vi "Init.vi"(8 "error in (no error)":errorcluster, 9 "SA Pin":string, 10 "Measurement Name":string) -> (0 "error out":errorcluster, 3 "GSM_ModAcc_out":refnum<class "GSM_ModAcc.lvclass">)   [LabVIEW 2016, in "SeqAuto Evaluations.lvlib" / "GSM_ModAcc.lvclass"]
uses:
  GSM_ModAcc.lvclass
  C:/Sequence Automation/Plugins/SeqAuto IEvaluation.lvlibp/SeqAuto IEvaluation.lvclass
  GSM_ModAcc.lvclass/GSM_ModAcc.ctl
  Plugins/SeqAuto IEvaluation.lvlibp/Write Measurement Name.vi
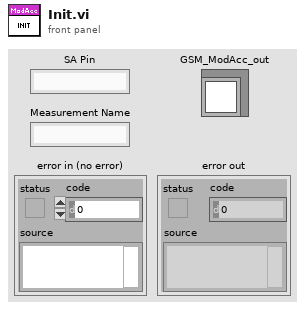
[diagram p1: front panel]
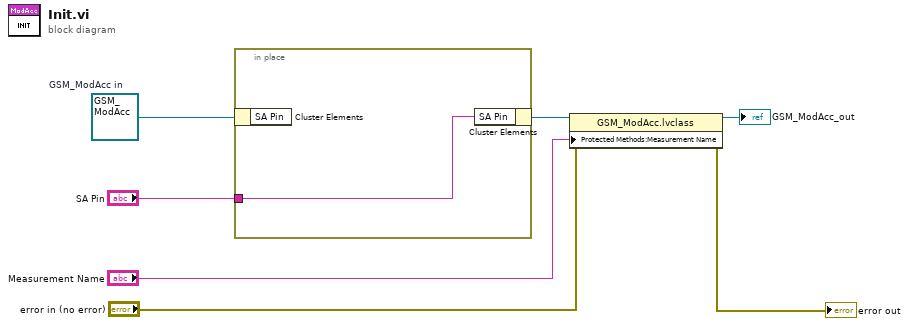
[diagram p0: block diagram]
diagram:
  w2 = refnum<class "GSM_ModAcc.lvclass"> refnum  # GSM_ModAcc in
  n1 = in-place {
    in-place-border: "SA Pin" -> [w8]
    n2 = in-place-cluster #1(w2) -> ()  [unwired: 1 out]
    n3 = in-place-cluster #1("SA Pin"=w8) -> (w4:refnum<class "GSM_ModAcc.lvclass">)
  }
  n4 = property class="GSM_ModAcc.lvclass"(reference=w4, error in="error in (no error)", "Protected Methods:Measurement Name"="Measurement Name") -> (reference out=→"GSM_ModAcc_out":refnum<class "GSM_ModAcc.lvclass">, error out=→"error out":errorcluster)
